vi "Close.vi"(8 "error in (no error)":errorcluster, 11 "Stream Upload Controller in":refnum<class "Stream Upload Controller.lvclass">) -> (0 "error out":errorcluster, 3 "Stream Upload Controller out":refnum<class "Stream Upload Controller.lvclass">)   [LabVIEW 2020, in "NI_SFTP.lvlib" / "Stream Upload Controller.lvclass"]
uses:
  <vilib>/net/SFTP/API/Support/Upload/Stream/Stream Upload Controller.lvclass
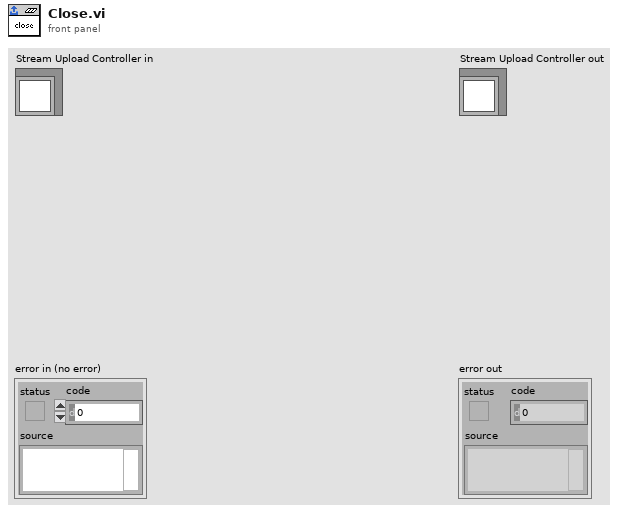
[diagram p1: front panel]
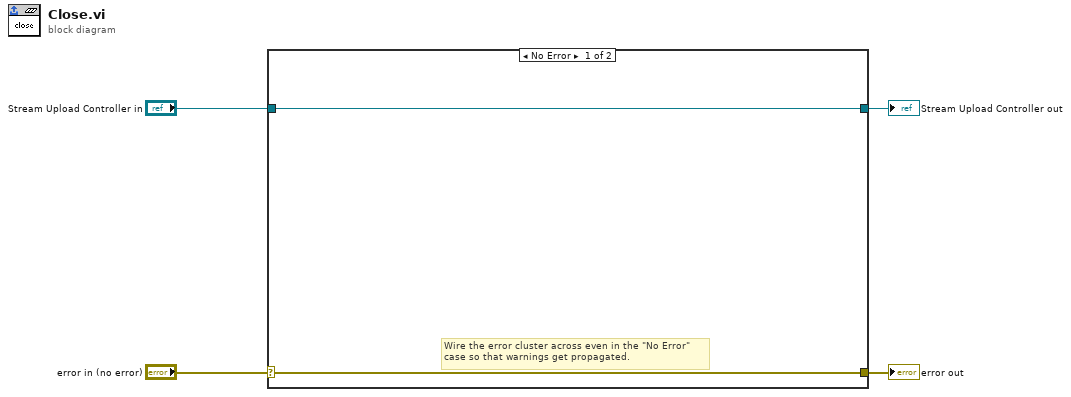
[diagram p0: block diagram]
diagram:
  n1 = case shown="No Error" "error in (no error)" {
    selector: "error in (no error)" -> [w5 w8]
    tunnel: [w5 w8] -> w3
    tunnel: [w6 w7] -> w1
    tunnel: "Stream Upload Controller in" -> [w6 w7]
    frame No Error {
      # "Wire the error cluster across even in the \"No Error\"\ncase so that warnings get propagated."
    }
    frame Error {
    }
  }
  "error out" <- w3
  "Stream Upload Controller out" <- w1
